vi "Orbit Hub.vi"   [LabVIEW 2025]
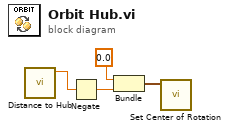
[diagram p0: block diagram]
diagram:
  n1 = call "Distance to Hub.vi"() -> ("Distance to Hub (ft)"=w2:dbl)  [unwired: 10 in, 1 out]
  n2 = Negate(x=w2) -> (-x=w3:dbl)
  n3 = Bundle(0.0, w3) -> (w1:cluster{dbl, dbl})  [unwired: 1 in]
  n4 = call "Set Center of Rotation.vi"("Center of Rotation"=w1) -> ()  [unwired: 10 in, 1 out]
